vi "subVIChecknavX.vi"() -> (0 "navX Device":T1={"Interface"={"Protocol"=enum."SERIAL", "Update Rate (4Hz-100Hz)"=4, "navX Open TypeDef"=variant}, "Notify Packet"=refnum, "Loop VI Refnum"=refnum, "Ready to Close Occurrence Refnum"=refnum} {"Interface"."Update Rate (4Hz-100Hz)" min=4 max=60 step=1}, 1 "Displacement navX":T3, 2 "Yaw":dbl, 3 "Roll":dbl, 4 "Fused Heading":dbl, 5 "Pitch":dbl, 6 "Heading":dbl)   [LabVIEW 2015]
uses:
  navX Library v2.lvlib
  TypeDefs/Z900_navX_ProtocolTypeDef.ctl
  TypeDefs/Z900_navX_ActionTypeDef.ctl
  TypeDefs/Z900_navX_NotifyPacketTypeDef.ctl
  TypeDefs/Z900_navX_DeviceTypeDef.ctl
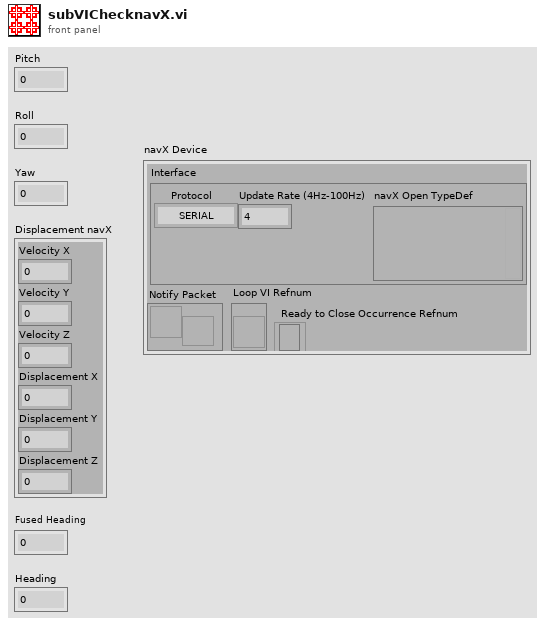
[diagram p1: front panel]
types:
  T1 = typedef "navX Library v2.lvlib/Z900_navX_DeviceTypeDef.ctl" = cluster{"Interface":cluster{"Protocol":T2, "Update Rate (4Hz-100Hz)":u8, "navX Open TypeDef":variant}, "Notify Packet":refnum<notifier>, "Loop VI Refnum":refnum<vi>, "Ready to Close Occurrence Refnum":refnum<k4>}
  T2 = typedef "navX Library v2.lvlib/Z900_navX_ProtocolTypeDef.ctl" = enum16{"SERIAL", "I2C", "SPI"}
  T3 = cluster{"Velocity X":dbl, "Velocity Y":dbl, "Velocity Z":dbl, "Displacement X":dbl, "Displacement Y":dbl, "Displacement Z":dbl}
  T4 = cluster{"Yaw":dbl, "Roll":dbl, "Pitch":dbl, "Heading":dbl, "Fused Heading":dbl}
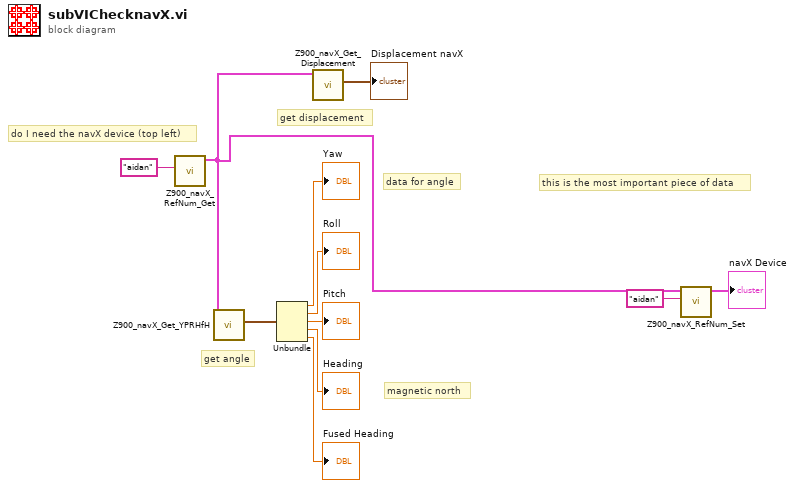
[diagram p0: block diagram]
diagram:
  # "do I need the navX device (top left)"
  # "magnetic north"
  # "this is the most important piece of data"
  # "data for angle"
  # "get angle"
  # "get displacement"
  n1 = call "Z900_navX_RefNum_Get.vi"("refnum name"="aidan") -> ("navX Device"=w3:T1)  [unwired: 9 in, 1 out]
  n2 = call "Z900_navX_Get_YPRHfH.vi"("navX Device"=w3) -> ("YRPHfH"=w6:T4)  [unwired: 7 in, 3 out]
  n3 = Unbundle(w6) -> ("Yaw"=→"Yaw":dbl, "Roll"=→"Roll":dbl, "Pitch"=→"Pitch":dbl, "Heading"=→"Heading":dbl, "Fused Heading"=→"Fused Heading":dbl)
  n4 = call "Z900_navX_Get_Displacement.vi"("navX Device"=w3) -> ("Displacement"=→"Displacement navX":T3)  [unwired: 7 in, 3 out]
  n5 = call "Z900_navX_RefNum_Set.vi"("refnum name"="aidan", "navX Device"=w3) -> ("navX Device"=→"navX Device":T1)  [unwired: 8 in, 1 out]
